vi "TrajectoryConfig_setKinematicsMecanumDrive.vi"(9 "MECA_DRIVE_KINEMATICS":T1={"FrontLeft"={"X"=0.0, "Y"=0.0}, "FrontRight"={"X"=0.0, "Y"=0.0}, "RearLeft"={"X"=0.0, "Y"=0.0}, "RearRight"={"X"=0.0, "Y"=0.0}, "InverseKinematics"=[[0.0, 1.0, -1.0, 0.0], [0.0, 1.0, 1.0, 0.0], [0.0, 1.0, 1.0, 0.0], [0.0, 1.0, -1.0, 0.0]], "ForwardKinematics"=[[0.0, 1.0, -1.0, 0.0], [0.0, 1.0, 1.0, 0.0], [0.0, 1.0, 1.0, 0.0], [0.0, 1.0, -1.0, 0.0]], "PrevCoR"={"X"=0.0, "Y"=0.0}} {"PrevCoR"."Y" format="%14.3f"; "PrevCoR"."X" format="%14.3f"; "RearRight"."Y" format="%14.3f"; "RearRight"."X" format="%14.3f"; "RearLeft"."Y" format="%14.3f"; "RearLeft"."X" format="%14.3f"; "FrontRight"."Y" format="%14.3f"; "FrontRight"."X" format="%14.3f"; "FrontLeft"."Y" format="%14.3f"; "FrontLeft"."X" format="%14.3f"}, 11 "inTRAJECTORY_CONFIG":T4 {"End Velocity" format="%20.4f"; "StartVelocity" format="%20.4f"; "Max Acceleration" format="%20.4f"; "MaxVelocity" format="%20.4f"}) -> (3 "outTRAJECTORY_CONFIG":T4 {"End Velocity" format="%20.4f"; "StartVelocity" format="%20.4f"; "Max Acceleration" format="%20.4f"; "MaxVelocity" format="%20.4f"})   [LabVIEW 2019, in "Trajectory_Library.lvlib"]
doc: "Adds and enabled a mecanum drive kinematics constraint to ensure that no wheel velocity of a mecanum drive goes above the max velocity. The TrajectoryConfiguration max velocity is used for the mecanum drive max individual wheel velocity.\n\nParameters:\n - MecanumDriveKinematics - The mecanum drive kinematics data structure\n - InTrajectoryConfig - The trajectory configuration data structure\n\nReturns:\n - OutTrajectoryConfig - Modified trajectory configuration data structure"
uses:
  Trajectory_Library.lvlib
  TypeDef/TRAJ_CONFIG.ctl
  TypeDef/MECA_DRIVE_KINEMATICS.ctl
  TypeDef/TRANSLATION2D.ctl
  <vilib>/Analysis/Matrix/Datatypes/RealMatrix.ctl
  <vilib>/Analysis/Matrix/NI_Matrix.lvlib
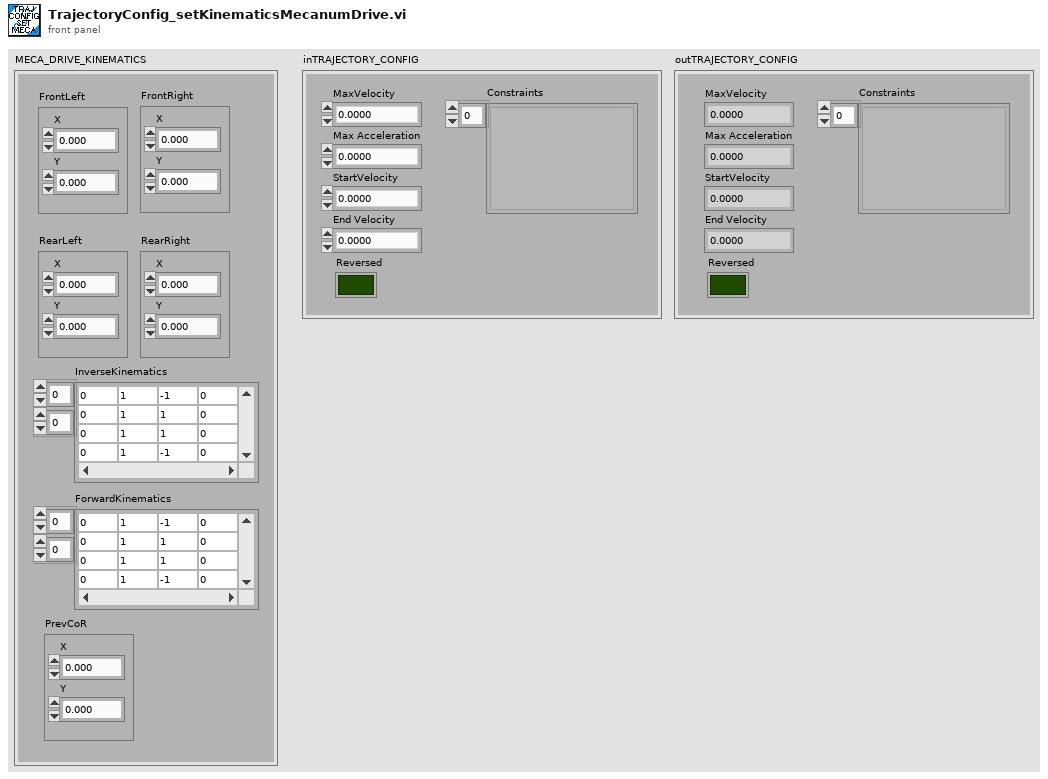
[diagram p1: front panel]
types:
  T1 = typedef "Trajectory_Library.lvlib/MECA_DRIVE_KINEMATICS.ctl" = cluster{"FrontLeft":T2, "FrontRight":T2, "RearLeft":T2, "RearRight":T2, "InverseKinematics":T3, "ForwardKinematics":T3, "PrevCoR":T2}
  T2 = typedef "Trajectory_Library.lvlib/TRANSLATION2D.ctl" = cluster{"X":dbl, "Y":dbl}
  T3 = typedef "NI_Matrix.lvlib/RealMatrix.ctl" = dbl[][]
  T4 = typedef "Trajectory_Library.lvlib/TRAJ_CONFIG.ctl" = cluster{"MaxVelocity":dbl, "Max Acceleration":dbl, "StartVelocity":dbl, "End Velocity":dbl, "Reversed":bool, "Constraints":variant[]}
  T5 = typedef "Trajectory_Library.lvlib/TRAJ_CONSTRAINT_MECA_DRIVE_KINEMATICS.ctl" = cluster{"Max Speed (M/S)":dbl, "MECA_DRIVE_KINEMATICS":T1}
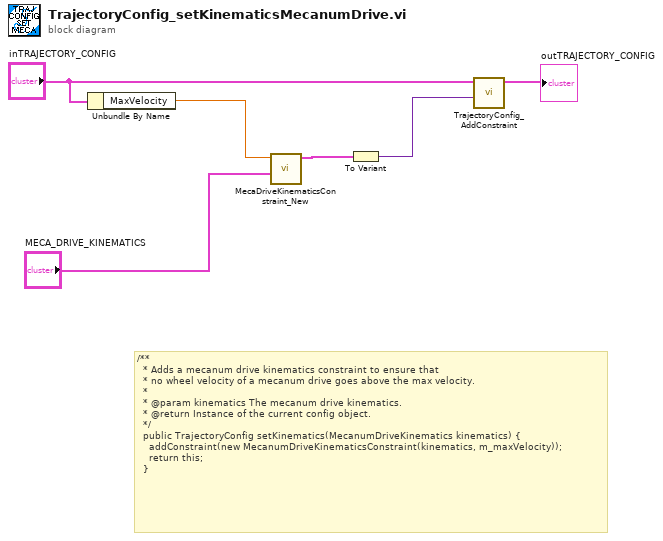
[diagram p0: block diagram]
diagram:
  # "/**\n  * Adds a mecanum drive kinematics constraint to ensure that\n  * no wheel velocity of a mecanum drive goes above the max velocity.\n  *\n  * @param kinematics The mecanum drive kinematics.\n  * @return Instance of the current config object.\n  */\n  public TrajectoryConfig setKinematics(MecanumDriveKinematics kinematics) {\n    addConstraint(new MecanumDriveKinematicsConstraint(kinematics, m_maxVelocity));\n    return this;\n  }"
  n1 = Unbundle By Name("inTRAJECTORY_CONFIG") -> ("MaxVelocity"=w6:dbl)
  n2 = call "MecaDriveKinematicsConstraint_New.vi"("MecanumKinematics"="MECA_DRIVE_KINEMATICS", "Max Speed (M/S)"=w6) -> ("MECANUM_DRIVE_KINE_CONSTRAINT"=w2:T5)  [unwired: 9 in]
  n3 = To Variant(anything=w2) -> (Variant=w4:variant)
  n4 = call "TrajectoryConfig_AddConstraint.vi"("Constraint"=w4, "inTRAJECTORY_CONFIG"="inTRAJECTORY_CONFIG") -> ("outTRAJECTORY_CONFIG"=→"outTRAJECTORY_CONFIG":T4)  [unwired: 9 in]
